vi "Main_UI.vi"(11 "Error_In":errorcluster) -> (15 "Error_Out":errorcluster)   [LabVIEW 2021]
doc: "This VI is the main VI which controls the flow of the game. does not have the front panel."
uses:
  Controls/State.ctl
types:
  T1 = typedef "State.ctl" = enum16{"Close", "Password_Popup", "Start_Popup", "Wizard_Msg", "Get_Name_DoB", "Lucky_Number", "Q-1", "Q-2", "Q-3", "Nature_of_the_Person"}
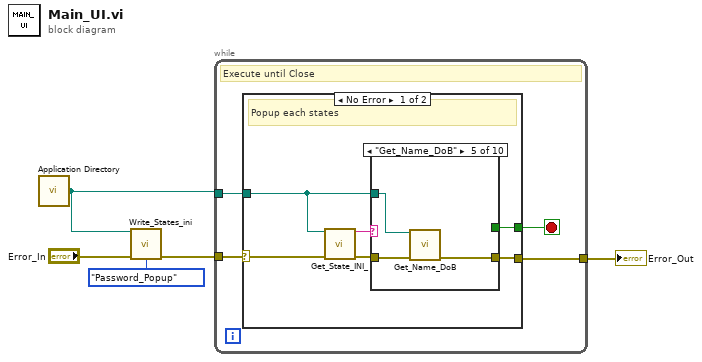
[diagram p0: block diagram]
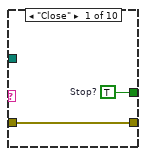
[diagram p2: hidden frame]
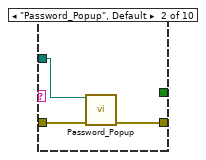
[diagram p3: hidden frame]
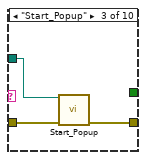
[diagram p4: hidden frame]
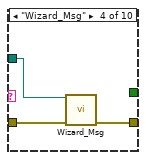
[diagram p5: hidden frame]
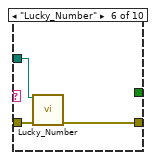
[diagram p6: hidden frame]
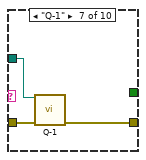
[diagram p7: hidden frame]
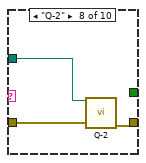
[diagram p8: hidden frame]
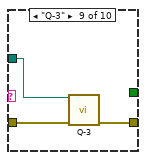
[diagram p9: hidden frame]
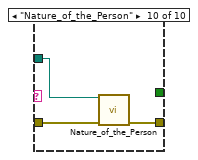
[diagram p10: hidden frame]
diagram:
  n1 = call <vilib>:"Application Directory.vi"() -> ("Application Directory"=w1:path)
  n2 = call "Write_States_ini.vi"("Application_Directory"=w1, "Error_In"="Error_In", "State"=State."Password_Popup") -> ("Error_Out"=w3:errorcluster)  [unwired: 12 in]
  n3 = while {
    tunnel: w3 -> [w9]
    tunnel: [w8] -> w5
    tunnel: w1 -> [w6]
    stop <- w7 stop-if-true
    # "Execute until Close"
    n4 = case shown="No Error" w9 {
      selector: w9 -> [w15 w45]
      tunnel: [w13 w45] -> w8
      tunnel: [w11 _] -> w7
      tunnel: w6 -> [w10 _]
      frame No Error {
        # "Popup each states"
        n5 = call "Get_State_INI_.vi"("Application_Directory"=w10, "Error_In"=w15) -> ("Data"=w14:string, "Error_Out"=w12:errorcluster)  [unwired: 12 in]
        n6 = case shown="\"Get_Name_DoB\"" w14 {
          tunnel: [w17 w19 w22 w25 w28 w31 w34 w37 w40 w43] -> w13
          tunnel: w12 -> [w17 w20 w23 w26 w29 w32 w35 w38 w41 w44]
          tunnel: [w16 _ _ _ _ _ _ _ _ _] -> w11
          tunnel: w10 -> [_ w18 w21 w24 w27 w30 w33 w36 w39 w42]
          frame "Close" {
            w16 = TRUE  # Stop?
            # "close game"
          }
          frame "Password_Popup", Default {
            n7 = call "Password_Popup.vi"("Application_Directory"=w18, "Error_In"=w20) -> ("Error_Out"=w19:errorcluster)  [unwired: 13 in]
          }
          frame "Start_Popup" {
            n8 = call "Start_Popup.vi"("Application_Directory"=w21, "Error_In"=w23) -> ("Error_Out"=w22:errorcluster)  [unwired: 13 in]
          }
          frame "Wizard_Msg" {
            n9 = call "Wizard_Msg.vi"("Application_Directory"=w24, "Error_In"=w26) -> ("Error_Out"=w25:errorcluster)  [unwired: 13 in]
          }
          frame "Get_Name_DoB" {
            n10 = call "Get_Name_DoB.vi"("Application_Directory"=w27, "Error_In"=w29) -> ("Error_Out"=w28:errorcluster)  [unwired: 11 in, 2 out]
          }
          frame "Lucky_Number" {
            n11 = call "Lucky_Number.vi"("Application_Directory"=w30, "Error_In"=w32) -> ("Error_Out"=w31:errorcluster)  [unwired: 13 in]
          }
          frame "Q-1" {
            n12 = call "Q-1.vi"("Application_Directory"=w33, "Error_In"=w35) -> ("Error_Out"=w34:errorcluster)  [unwired: 13 in]
          }
          frame "Q-2" {
            n13 = call "Q-2.vi"("Application_Directory"=w36, "Error_In"=w38) -> ("Error_Out"=w37:errorcluster)  [unwired: 13 in]
          }
          frame "Q-3" {
            n14 = call "Q-3.vi"("Application_Directory"=w39, "Error_In"=w41) -> ("Error_Out"=w40:errorcluster)  [unwired: 13 in]
          }
          frame "Nature_of_the_Person" {
            n15 = call "Nature_of_the_Person.vi"("Application_Directory"=w42, "Error_In"=w44) -> ("Error_Out"=w43:errorcluster)  [unwired: 13 in]
          }
        }
      }
      frame Error {
      }
    }
  }
  "Error_Out" <- w5
